vi "Create Window.vi"(8 "error in (no error)":errorcluster, 10 "Fs (Hz)":dbl, 11 "Gate in":refnum<class "Gate.lvclass">) -> (0 "error out":errorcluster, 2 "Window":dbl[](array[numeric]), 3 "Gate out":refnum<class "Gate.lvclass">)   [LabVIEW 2020, in "Gate.lvclass"]
uses:
  Gate.lvclass
  Gate.lvclass/Gate.ctl
  <vilib>/Analysis/1siggen.llb/Ramp Pattern by Samples.vi
  f9597422-770a-4678-bdca-162a0152deaa.vi
  <vilib>/Analysis/NI_AALBase.lvlib
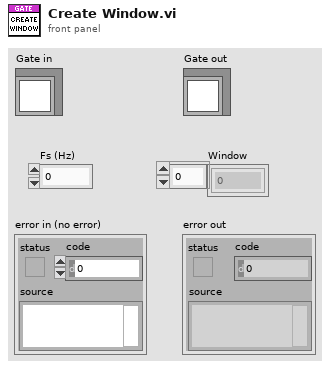
[diagram p1: front panel]
types:
  T1 = typedef "Gate.lvclass/Shape.ctl" = enum16{"OFF", "Rectangle", "Sine-squared", "Trapezoid"}
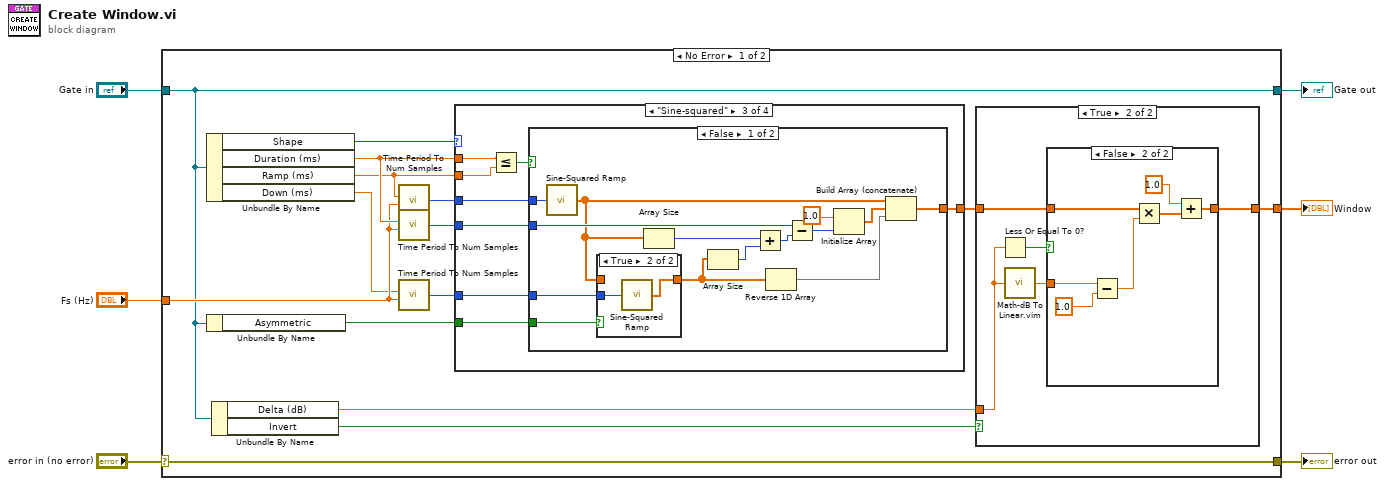
[diagram p0: block diagram]
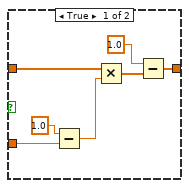
[diagram p3: hidden frame]
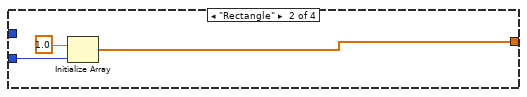
[diagram p5: hidden frame]
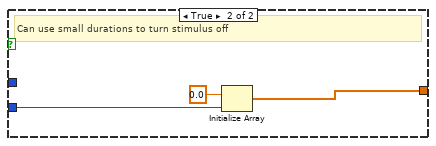
[diagram p7: hidden frame]
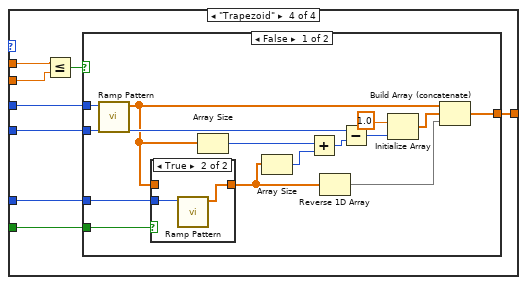
[diagram p8: hidden frame]
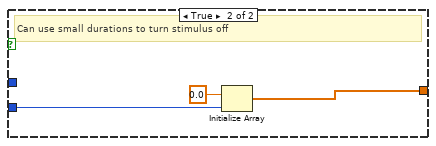
[diagram p10: hidden frame]
diagram:
  n1 = case shown="No Error" "error in (no error)" {
    selector: "error in (no error)" -> [w21 w102]
    tunnel: [w21 w102] -> w5
    tunnel: [w11 w101] -> w3
    tunnel: "Gate in" -> [w11 w101]
    tunnel: "Fs (Hz)" -> [w15 _]
    tunnel: [w8 _] -> w1
    frame No Error {
      n2 = Unbundle By Name(w11) -> ("Shape"=w20:T1, "Duration (ms)"=w18:dbl, "Ramp (ms)"=w17:dbl, "Down (ms)"=w14:dbl)
      n3 = Unbundle By Name(w11) -> ("Asymmetric"=w13:bool)
      n4 = Unbundle By Name(w11) -> ("Delta (dB)"=w7:dbl, "Invert"=w9:bool)
      n5 = call "Time Period To Num Samples.vi"("Duration (ms)"=w17, "Sampling rate (Hz)"=w15) -> ("Samples"=w16:i32)  [unwired: 5 in]
      n6 = call "Time Period To Num Samples.vi"("Duration (ms)"=w18, "Sampling rate (Hz)"=w15) -> ("Samples"=w19:i32)  [unwired: 5 in]
      n7 = call "Time Period To Num Samples.vi"("Duration (ms)"=w14, "Sampling rate (Hz)"=w15) -> ("Samples"=w12:i32)  [unwired: 5 in]
      n8 = case shown="\"Sine-squared\"" w20 {
        tunnel: w19 -> [_ w44 w49 w77]
        tunnel: [_ w42 w48 w76] -> w10
        tunnel: w18 -> [_ _ w52 w80]
        tunnel: w17 -> [_ _ w51 w79]
        tunnel: w16 -> [_ _ w47 w75]
        tunnel: w13 -> [_ _ w46 w74]
        tunnel: w12 -> [_ _ w45 w73]
        frame "OFF", Default {
        }
        frame "Rectangle" {
          n9 = Initialize Array(1.0, w44) -> (w42:dbl[])
        }
        frame "Sine-squared" {
          n10 = Less Or Equal?(x=w52, y=w51) -> (x <= y?=w50:bool)
          n11 = case shown="False" w50 {
            tunnel: w49 -> [w64 w71]
            tunnel: [w60 w70] -> w48
            tunnel: w47 -> [w61 _]
            tunnel: w46 -> [w59 _]
            tunnel: w45 -> [w58 _]
            frame False {
              n12 = call "Sine-Squared Ramp.vi"("Samples"=w61) -> ("Sine-squared ramp"=w57:dbl[])  [unwired: 14 in]
              n13 = case shown="True" w59 {
                tunnel: w57 -> [w67 _]
                tunnel: [w67 w68] -> w54
                tunnel: w58 -> [_ w69]
                frame False {
                }
                frame True {
                  n14 = call "Sine-Squared Ramp.vi"("Samples"=w69) -> ("Sine-squared ramp"=w68:dbl[])  [unwired: 14 in]
                }
              }
              n15 = Array Size(array=w57) -> (size(s)=w56:i32)
              n16 = Array Size(array=w54) -> (size(s)=w53:i32)
              n17 = Add(x=w56, y=w53) -> (x+y=w55:i32)
              n18 = Reverse 1D Array(array=w54) -> (reversed array=w66:dbl[])
              n19 = Subtract(x=w64, y=w55) -> (x-y=w63:i32)
              n20 = Initialize Array(1.0, w63) -> (w65:dbl[])
              n21 = Build Array (concatenate)(w57, w65, w66) -> (w60:dbl[])
            }
            frame True {
              # "Can use small durations to turn stimulus off"
              n22 = Initialize Array(0.0, w71) -> (w70:dbl[])
            }
          }
        }
        frame "Trapezoid" {
          n23 = Less Or Equal?(x=w80, y=w79) -> (x <= y?=w78:bool)
          n24 = case shown="False" w78 {
            tunnel: w77 -> [w92 w99]
            tunnel: [w89 w98] -> w76
            tunnel: w75 -> [w82 _]
            tunnel: w74 -> [w88 _]
            tunnel: w73 -> [w87 _]
            frame False {
              n25 = call-poly <vilib>:"Ramp Pattern.vi"("samples"=w82) -> ("Ramp Pattern"=w81:dbl[])  [unwired: 9 in, 1 out]
              n26 = case shown="True" w88 {
                tunnel: w81 -> [w95 _]
                tunnel: [w95 w96] -> w84
                tunnel: w87 -> [_ w97]
                frame False {
                }
                frame True {
                  n27 = call-poly <vilib>:"Ramp Pattern.vi"("samples"=w97) -> ("Ramp Pattern"=w96:dbl[])  [unwired: 9 in, 1 out]
                }
              }
              n28 = Array Size(array=w81) -> (size(s)=w86:i32)
              n29 = Array Size(array=w84) -> (size(s)=w83:i32)
              n30 = Add(x=w86, y=w83) -> (x+y=w85:i32)
              n31 = Reverse 1D Array(array=w84) -> (reversed array=w94:dbl[])
              n32 = Subtract(x=w92, y=w85) -> (x-y=w91:i32)
              n33 = Initialize Array(1.0, w91) -> (w93:dbl[])
              n34 = Build Array (concatenate)(w81, w93, w94) -> (w89:dbl[])
            }
            frame True {
              # "Can use small durations to turn stimulus off"
              n35 = Initialize Array(0.0, w99) -> (w98:dbl[])
            }
          }
        }
      }
      n36 = case shown="True" w9 {
        tunnel: w10 -> [w22 w27]
        tunnel: [w22 w23] -> w8
        tunnel: w7 -> [_ w26]
        frame False {
        }
        frame True {
          n37 = Less Or Equal To 0?(x=w26) -> (x <= 0?=w24:bool)
          n38 = call "Math-dB To Linear.vim"("dB"=w26) -> ("linear"=w25:dbl)
          n39 = case shown="False" w24 {
            tunnel: w27 -> [w30 w37]
            tunnel: w25 -> [w32 w39]
            tunnel: [w28 w35] -> w23
            frame True {
              n40 = Subtract(x=1.0, y=w32) -> (x-y=w29:dbl)
              n41 = Multiply(x=w30, y=w29) -> (x*y=w33:dbl[])
              n42 = Subtract(x=1.0, y=w33) -> (x-y=w28:dbl[])
            }
            frame False {
              n43 = Subtract(x=w39, y=1.0 ("x")) -> (x-y=w36:dbl)
              n44 = Multiply(x=w37, y=w36) -> (x*y=w40:dbl[])
              n45 = Add(x=1.0, y=w40) -> (x+y=w35:dbl[])
            }
          }
        }
      }
    }
    frame Error {
    }
  }
  "error out" <- w5
  "Gate out" <- w3
  "Window" <- w1
